vi "Generate Waveform.vi"(0 "Downsampling":dbl, 1 "Data Period (s)":dbl, 2 "Data":dbl[][](array[numeric]), 3 "Plot names":string[](array[string]), 4 "Time Stamp":timestamp) -> (5 "Downsampled data":waveform(dbl)[](array[waveform]), 6 "Non downsampled waveform":waveform(dbl)[](array[waveform]))   [LabVIEW 2014]
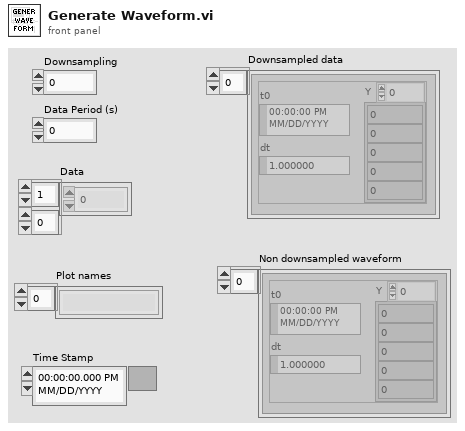
[diagram p1: front panel]
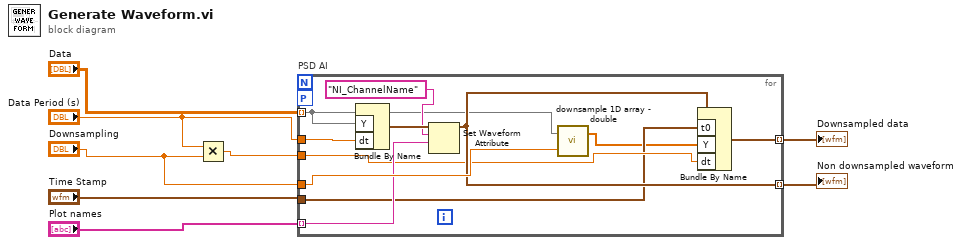
[diagram p0: block diagram]
diagram:
  n1 = Multiply(x="Data Period (s)", y="Downsampling") -> (x*y=w5:dbl)
  n2 = for "PSD AI" {
    tunnel: [w19] -> w2 mode=indexing
    tunnel: "Time Stamp" -> [w12]
    tunnel: "Downsampling" -> [w18]
    tunnel: "Data" -> [w9] mode=indexing
    tunnel: "Data Period (s)" -> [w16]
    tunnel: "Plot names" -> [w15] mode=indexing
    tunnel: [w14] -> w1 mode=indexing
    tunnel: w5 -> [w13]
    workers-P: _ -> [_]
    n3 = Bundle By Name("Y"=w9, "dt"=w16) -> (w17:waveform(dbl))  [unwired: 1 out]
    n4 = Set Waveform Attribute(5:w15, 6:"NI_ChannelName" ("name"), 7:w17) -> (3:w14:waveform(dbl))  [unwired: 1 in, 2 out]
    n5 = call "downsample 1D array - double.vi"("Ave N"=w18, "Array In"=w9) -> ("Array Out"=w10:dbl[])  [unwired: 1 out]
    n6 = Bundle By Name(cluster=w14, "t0"=w12, "Y"=w10, "dt"=w13) -> (w19:waveform(dbl))
  }
  "Downsampled data" <- w2
  "Non downsampled waveform" <- w1
